vi "destroy.vi"(8 "error in":errorcluster, 11 "TLS HTTP server in":refnum<class "TLS HTTP server.lvclass">) -> (0 "error out":errorcluster)   [LabVIEW 2016, in "TLS HTTP server.lvclass"]
uses:
  TLS HTTP server.lvclass
  TLS HTTP server.lvclass/TLS HTTP server.ctl
  HTTP server/Basic HTTP server.lvclass
  lvlibtls/server/lvlibretls server listener.lvclass
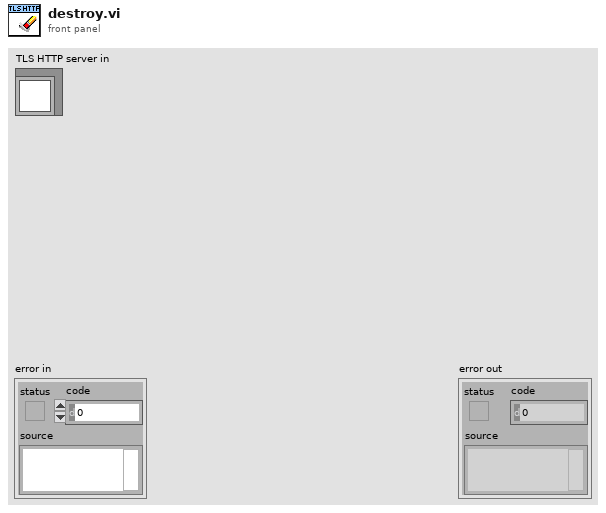
[diagram p1: front panel]
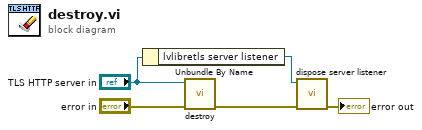
[diagram p0: block diagram]
diagram:
  n1 = Unbundle By Name("TLS HTTP server in") -> ("lvlibretls server listener"=w4:refnum<class "lvlibretls server listener.lvclass">)
  n2 = call-parent "destroy.vi"("error in"="error in", "Basic HTTP server in"="TLS HTTP server in") -> ("error out"=w2:errorcluster)  [unwired: 9 in]
  n3 = call "dispose server listener.vi"("error in"=w2, "lvlibretls server listener in"=w4) -> ("error out"=→"error out":errorcluster)  [unwired: 9 in]
